vi "PKG_IMC_Close.vi"(11 "Handle":u32) -> (2 "function return":i32, 3 "Handle out":u32)   [LabVIEW 2018, in "IMC_Pkg4xxx.lvlib"]
doc: "PKG_IMC_Close (IMC_HANDLE Handle);"
uses:
  IMC_Pkg4xxx.lvlib
  IMC_Pkg4xxx.dll
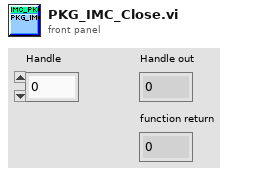
[diagram p1: front panel]
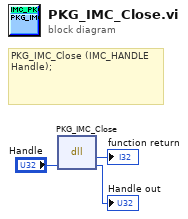
[diagram p0: block diagram]
diagram:
  # "PKG_IMC_Close (IMC_HANDLE Handle);"
  n1 = dll-call lib="PTH2\\abs D做的项目航天测量驱动电机IMCAppincLabview32\nIMC_Pkg4xxx.*" fn="PKG_IMC_Close"("Handle"="Handle") -> (→"function return":i32, "Handle"=→"Handle out":u32)  [unwired: 3 in, 2 out]
